vi "User Interface.vi"(8 "error in (no error)":errorcluster, 11 "User Interface in":refnum<class "User Interface.lvclass">) -> (0 "error out":errorcluster, 3 "User Interface out":refnum<class "User Interface.lvclass">)   [LabVIEW 2017, in "UDP Transceiver.lvlib" / "UDP Thread User Interface.lvclass"]
uses:
  UDP Thread User Interface.lvclass
  DSF Core.lvlibp/Classes/User Interface/User Interface.lvclass
  Configuration/Thread/UDP Thread Configuration.lvclass
  C:/Git/DSF/Components/DSF Core.lvlibp/Classes/Configuration/Configuration.lvclass
panel:
  in  "Local Address":string
  in  "Local Port":u16
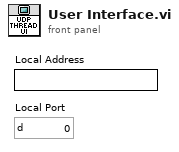
[diagram p1: front panel]
types:
  T1 = typedef "UDP Transceiver.lvlib/UDP Thread Configuration.lvclass/Thread Settings.ctl" = cluster{"local port":u16, "local address":u32}
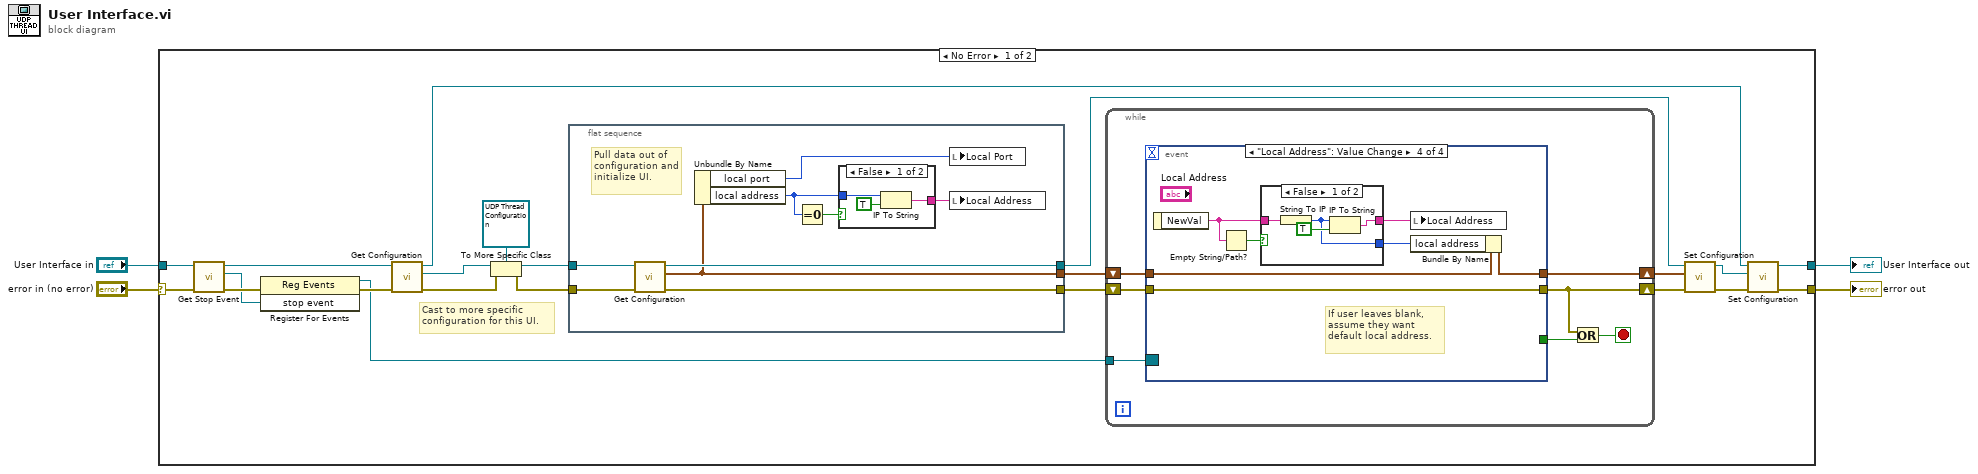
[diagram p0: block diagram]
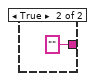
[diagram p2: hidden frame]
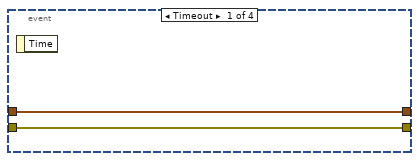
[diagram p3: hidden frame]
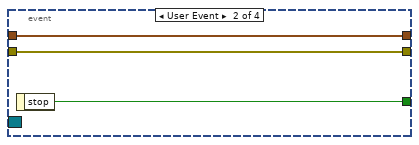
[diagram p4: hidden frame]
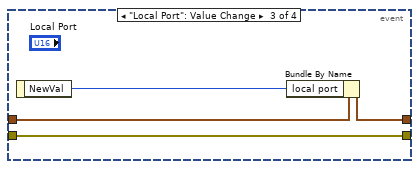
[diagram p5: hidden frame]
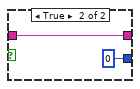
[diagram p6: hidden frame]
diagram:
  n1 = case shown="No Error" "error in (no error)" {
    selector: "error in (no error)" -> [w23 w70]
    tunnel: [w14 w70] -> w4
    tunnel: "User Interface in" -> [w22 w69]
    tunnel: [w13 w69] -> w1
    frame No Error {
      # "Cast to more specific configuration for this UI."
      n2 = call "Get Stop Event.vi"("error in (no error)"=w23, "User Interface in"=w22) -> ("error out"=w21:errorcluster, "stop event"=w20:refnum<user-event>, "User Interface out"=w19:refnum<class "User Interface.lvclass">)  [unwired: 7 in]
      n3 = register-events(error in=w21, w20) -> (reference out=w17:refnum<event-registration>, error out=w18:errorcluster)  [unwired: 1 in]
      n4 = call "Get Configuration.vi"("error in (no error)"=w18, "User Interface in"=w19) -> ("error out"=w16:errorcluster, "configuration"=w15:refnum<class "Configuration.lvclass">, "User Interface out"=w12:refnum<class "User Interface.lvclass">)  [unwired: 7 in]
      n5 = To More Specific Class(target class=refnum<class "UDP Thread Configuration.lvclass"> refnum ("DSF Core.lvlib:DSF UDP Thread Configuration"), reference=w15, error in=w16) -> (specific class reference=w26:refnum<class "UDP Thread Configuration.lvclass">, error out=w24:errorcluster)
      n6 = flat-sequence {
        tunnel: [w33] -> w25
        tunnel: w24 -> [w35]
        tunnel: w26 -> [w34]
        tunnel: [w30] -> w6
        tunnel: [w27] -> w10
        frame #0 {
          # "Pull data out of configuration and initialize UI."
          n7 = call "Get Configuration.vi"("error in (no error)"=w35, "DSF UDP Thread Configuration in"=w34) -> ("error out"=w33:errorcluster, "thread settings"=w27:T1, "DSF UDP Thread Configuration out"=w30:refnum<class "UDP Thread Configuration.lvclass">)  [unwired: 7 in]
          n8 = Unbundle By Name(w27) -> ("local port"=w32:u16, "local address"=w29:u32)
          n9 = Equal To 0?(x=w29) -> (x = 0?=w28:bool)
          n10 = case shown="False" w28 {
            tunnel: [w38 "" ("name")] -> w31
            tunnel: w29 -> [w37 _]
            frame False {
              n11 = IP To String(1:TRUE ("dot notation? (F)"), 2:w37) -> (0:w38:string)
            }
            frame True {
            }
          }
          n12 = local write "Local Port"(w32) -> ()
          n13 = local write "Local Address"(w31) -> ()
        }
      }
      n14 = while {
        tunnel: w17 -> [w46]
        shift-right: [w44] -> w9
        shift-left: w25 -> [w45]
        shift-right: [w40] -> w7
        shift-left: w10 -> [w41]
        stop <- w43 stop-if-true
        n15 = event shown="[3] \"Local Address\": Value Change" {
          selector: w46 -> [_ _ _ _]
          dyn-events: _ -> [_ _ _ _]
          timeout: _ -> [_ _ _ _]
          tunnel: [_ w50 _ _] -> w42
          tunnel: w45 -> [w48 w51 w55 w59]
          tunnel: [w48 w51 w55 w59] -> w44
          tunnel: w41 -> [w47 w49 w54 w60]
          tunnel: [w47 w49 w53 w62] -> w40
          event Timeout {
            n16 = event-data() -> ()  [unwired: 1 in, 1 out]
          }
          event User Event {
            n17 = event-data() -> ("stop"=w50:bool)  [unwired: 1 in]
          }
          event "Local Port": Value Change {
            n18 = event-data() -> ("NewVal"=w52:u16)  [unwired: 1 in]
            n19 = Bundle By Name(cluster=w54, "local port"=w52) -> (w53:T1)
          }
          event "Local Address": Value Change {
            # "If user leaves blank, assume they want default local address."
            n20 = event-data() -> ("NewVal"=w57:string)  [unwired: 1 in]
            n21 = Empty String/Path?(string/path=w57) -> (empty?=w58:bool)
            n22 = case shown="False" w58 {
              tunnel: [w66 w67] -> w61
              tunnel: w57 -> [w65 w67]
              tunnel: [w63 u32 0] -> w56
              frame False {
                n23 = String To IP(1:w65) -> (0:w63:u32)
                n24 = IP To String(1:TRUE ("dot notation? (F)"), 2:w63) -> (0:w66:string)
              }
              frame True {
              }
            }
            n25 = local write "Local Address"(w61) -> ()
            n26 = Bundle By Name(cluster=w60, "local address"=w56) -> (w62:T1)
          }
        }
        n27 = Or(x=w44, y=w42) -> (x .or. y?=w43:bool)
      }
      n28 = call "Set Configuration.vi"("error in (no error)"=w9, "thread settings"=w7, "DSF UDP Thread Configuration in"=w6) -> ("error out"=w8:errorcluster, "DSF UDP Thread Configuration out"=w5:refnum<class "UDP Thread Configuration.lvclass">)  [unwired: 7 in]
      n29 = call "Set Configuration.vi"("error in (no error)"=w8, "configuration"=w5, "User Interface in"=w12) -> ("error out"=w14:errorcluster, "User Interface out"=w13:refnum<class "User Interface.lvclass">)  [unwired: 7 in]
    }
    frame Error {
    }
  }
  "error out" <- w4
  "User Interface out" <- w1
